vi "DataPacker_SerializeBundle.vi"(8 "error in (no error)":errorcluster, 11 "DataPacker in":refnum<class "DataPacker.lvclass">) -> (0 "error out":errorcluster, 1 "Length of \nData bundle":i32, 2 "SerialisedData":string, 3 "DataPacker out":refnum<class "DataPacker.lvclass">, 4 "MIDAS Buffer \n[for this PC] \nUsage (%)":dbl(knob) scale=0.0..100.0)   [LabVIEW 2018, in "feGEM DataPacker.lvlib" / "DataPacker.lvclass"]
uses:
  DataPacker.lvclass
  DataPacker.lvclass/DataPacker.ctl
  DataStructures/GEM_BANK_ARRAY.lvclass/GEM_BANK_ARRAY.ctl
  DataStructures/GEM_BANK_ARRAY.lvclass
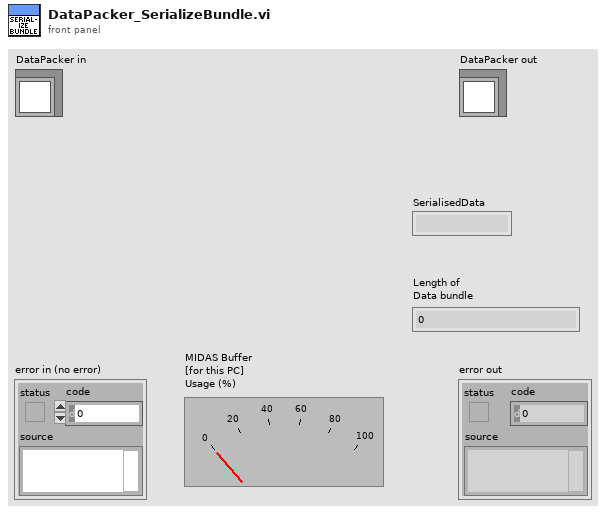
[diagram p1: front panel]
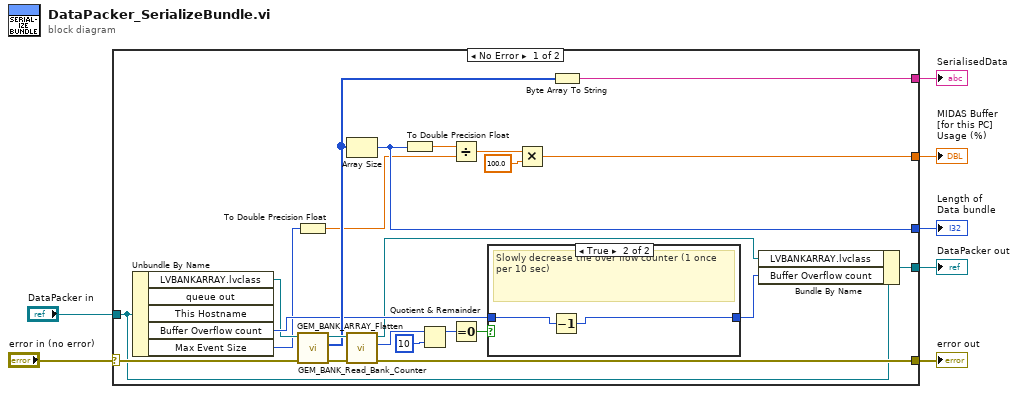
[diagram p0: block diagram]
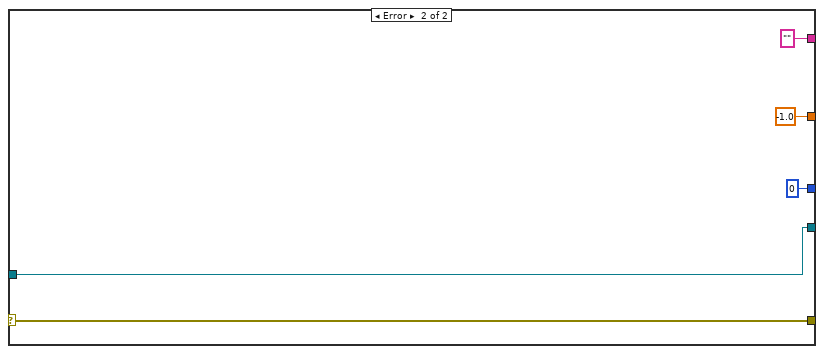
[diagram p3: hidden frame]
diagram:
  n1 = case shown="No Error" "error in (no error)" {
    selector: "error in (no error)" -> [w22 w38]
    tunnel: [w20 w38] -> w6
    tunnel: [w16 w37] -> w4
    tunnel: "DataPacker in" -> [w17 w37]
    tunnel: [w8 -1.0] -> w3
    tunnel: [w15 "" ("string")] -> w2
    tunnel: [w14 0] -> w1
    frame No Error {
      n2 = Unbundle By Name(w17) -> ("LVBANKARRAY.lvclass"=w21:refnum<class "GEM_BANK_ARRAY.lvclass">, "Buffer Overflow count"=w23:u32, "Max Event Size"=w9:u32)  [unwired: 2 out]
      n3 = To Double Precision Float(number=w9) -> (double precision float=w12:dbl)
      n4 = call "GEM_BANK_ARRAY_Flatten.vi"("error in (no error)"=w22, "LVBANKARRAY in"=w21) -> ("error out"=w27:errorcluster, "Array"=w25:u8[], "LVBANKARRAY out"=w26:refnum<class "GEM_BANK_ARRAY.lvclass">)  [unwired: 7 in]
      n5 = Array Size(array=w25) -> (size(s)=w14:i32)
      n6 = call "GEM_BANK_Read_Bank_Counter.vi"("error in (no error)"=w27, "GEM_BANK_ARRAY in"=w26) -> ("error out"=w20:errorcluster, "Bank Counter"=w28:u32, "GEM_BANK_ARRAY out"=w19:refnum<class "GEM_BANK_ARRAY.lvclass">)  [unwired: 7 in]
      n7 = To Double Precision Float(number=w14) -> (double precision float=w11:dbl)
      n8 = Quotient & Remainder(x=w28, y=u32 10) -> (x-y*floor(x/y)=w29:u32)  [unwired: 1 out]
      n9 = Divide(x=w11, y=w12) -> (x/y=w13:dbl)
      n10 = Equal To 0?(x=w29) -> (x = 0?=w30:bool)
      n11 = case shown="True" w30 {
        tunnel: [w31 w33] -> w18
        tunnel: w23 -> [w31 w32]
        frame False {
        }
        frame True {
          # "Slowly decrease the over flow counter (1 once per 10 sec)"
          n12 = Decrement(x=w32) -> (x-1=w33:u32)
        }
      }
      n13 = Multiply(x=w13, y=100.0) -> (x*y=w8:dbl)
      n14 = Byte Array To String(unsigned byte array=w25) -> (string=w15:string)
      n15 = Bundle By Name(cluster=w17, "LVBANKARRAY.lvclass"=w19, "Buffer Overflow count"=w18) -> (w16:refnum<class "DataPacker.lvclass">)
    }
    frame Error {
    }
  }
  "error out" <- w6
  "DataPacker out" <- w4
  "MIDAS Buffer \n[for this PC] \nUsage (%)" <- w3
  "SerialisedData" <- w2
  "Length of \nData bundle" <- w1
